vi "Autonomous Independent.vi"   [LabVIEW 2019]
doc: "This VI is called when autonomous begins, and will automatically be terminated when autonomous ends. You can carry out timed or sensor driven robot movement independently without needing to return to the caller."
uses:
  <vilib>/Rock Robotics/WPI/Utilities/WPI_GetSetVariantRefNum.vi
  Robot Global Data.vi
  <vilib>/Rock Robotics/Network Tables/NT Write Number.vi
  <vilib>/Rock Robotics/WPI/RobotDrive/WPI_RobotDriveArcadeDrive_Standard(NoSaturation).vi
  <vilib>/Rock Robotics/Network Tables/NT Write Numeric Array.vi
  <vilib>/Rock Robotics/Network Tables/NT Read String.vi
panel:
  # "Be sure to right-click and choose Data Operations>>Make Current Value default if you want to save the array values with the VI"
types:
  T1 = typedef "WPI_JoystickDevRef.ctl" = cluster{"Device":T2}
  T2 = typedef "WPI_JoystickDeviceEnum.ctl" = enum16{"USB 0", "USB 1", "USB 2", "USB 3", "USB 4", "USB 5"}
  T3 = typedef "WPI_RobotDriveDevRef.ctl" = cluster{"DevStatus":errorcluster, "Motors[]":T4[], "Square Inputs":bool, "Max Output":dbl}
  T4 = typedef "WPI_MotorControlDeviceRef.ctl" = cluster{"DeviceStatus":errorcluster, "Type":T5, "PWM":cluster{"PWM Channel":T6, "DeadBand":T7}, "CAN":cluster{"Device Number":u8, "SetOutput VI Ref":variant, "GetOutput VI Ref":variant, "Enable VI Ref":variant, "Disable VI Ref":variant, "Data":variant}, "Invert":bool, "DIO PWM":cluster{"PWM \"Enable\" Channel":T6, "DIOChannel":T8, "PWM Rate":dbl}}
  T5 = typedef "WPI_MotorControlType.ctl" = enum16{"PWM", "CAN", "DIO PWM"}
  T6 = typedef "FPGA_DIOPWMChannel.ctl" = enum8{"PWM 0", "PWM 1", "PWM 2", "PWM 3", "PWM 4", "PWM 5", "PWM 6", "PWM 7", "PWM 8", "PWM 9", "PWM MXP 0", "PWM MXP 1", "PWM MXP 2", "PWM MXP 3", "PWM MXP 4", "PWM MXP 5", "PWM MXP 6", "PWM MXP 7", "PWM MXP 8", "PWM MXP 9", "Invalid"}
  T7 = typedef "WPI_PWMDeadband.ctl" = cluster{"Name":string, "maxPositivePwm":i32, "minPositivePwm":i32, "centerPwm":i32, "maxNegativePwm":i32, "minNegativePwm":i32, "angularRange":u16}
  T8 = typedef "FPGA_DIOChannel.ctl" = enum8{"DIO 0", "DIO 1", "DIO 2", "DIO 3", "DIO 4", "DIO 5", "DIO 6", "DIO 7", "DIO 8", "DIO 9", "DIO MXP 0", "DIO MXP 1", "DIO MXP 2", "DIO MXP 3", "DIO MXP 4", "DIO MXP 5", "DIO MXP 6", "DIO MXP 7", "DIO MXP 8", "DIO MXP 9", "DIO MXP 10", "DIO MXP 11", "DIO MXP 12", "DIO MXP 13", "DIO MXP 14", "DIO MXP 15", "SPI Port CS1", "SPI Port CS2", "SPI Port CS3", "SPI Port MISO", "SPI Port MOSI", "Invalid"}
  T9 = typedef "WPI_ServoDeviceRef.ctl" = cluster{"DeviceStatus":errorcluster, "PWM Channel":T6, "DeadBand":T7}
  T10 = cluster{"RobotDriveDevRef":T3, "MotorControlDevRef":T4, "MotorControlDevRef":T4, "ServoDeviceRef":T9, "MotorControlDevRef":T4, "Distance":dbl}
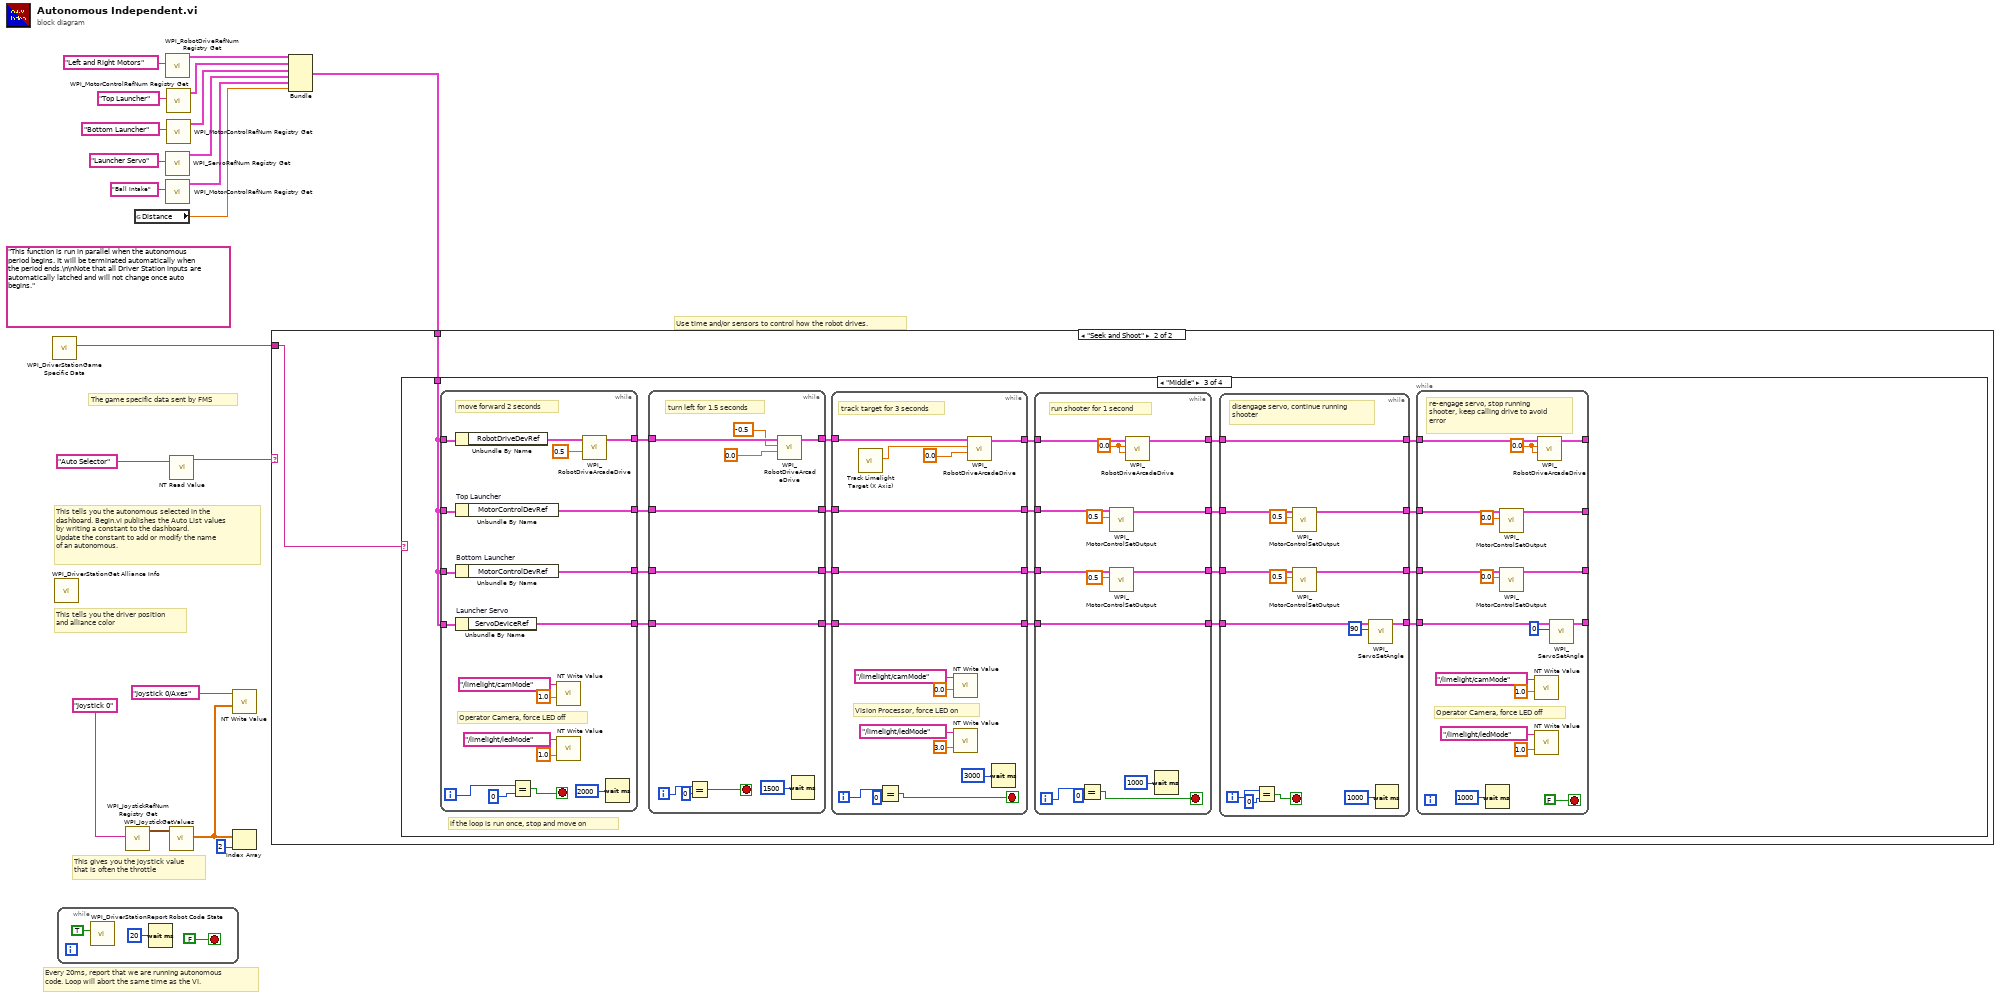
[diagram p0: block diagram]
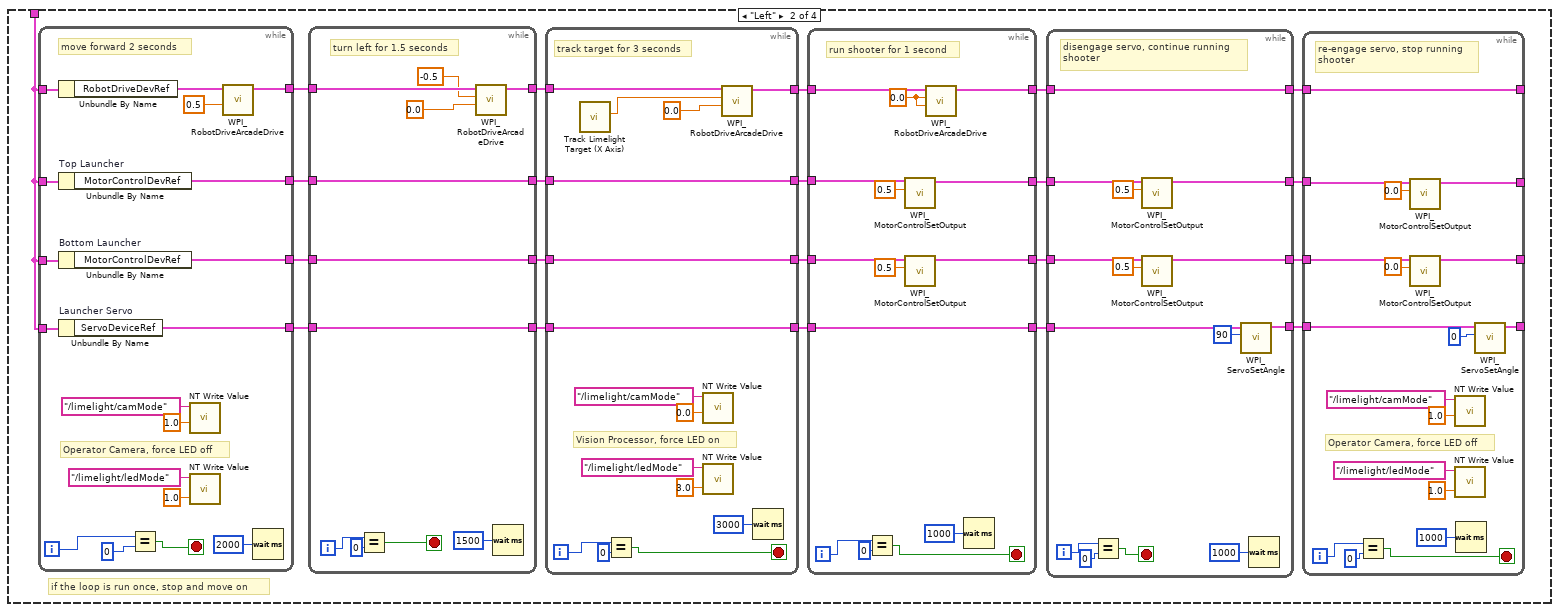
[diagram p4: hidden frame]
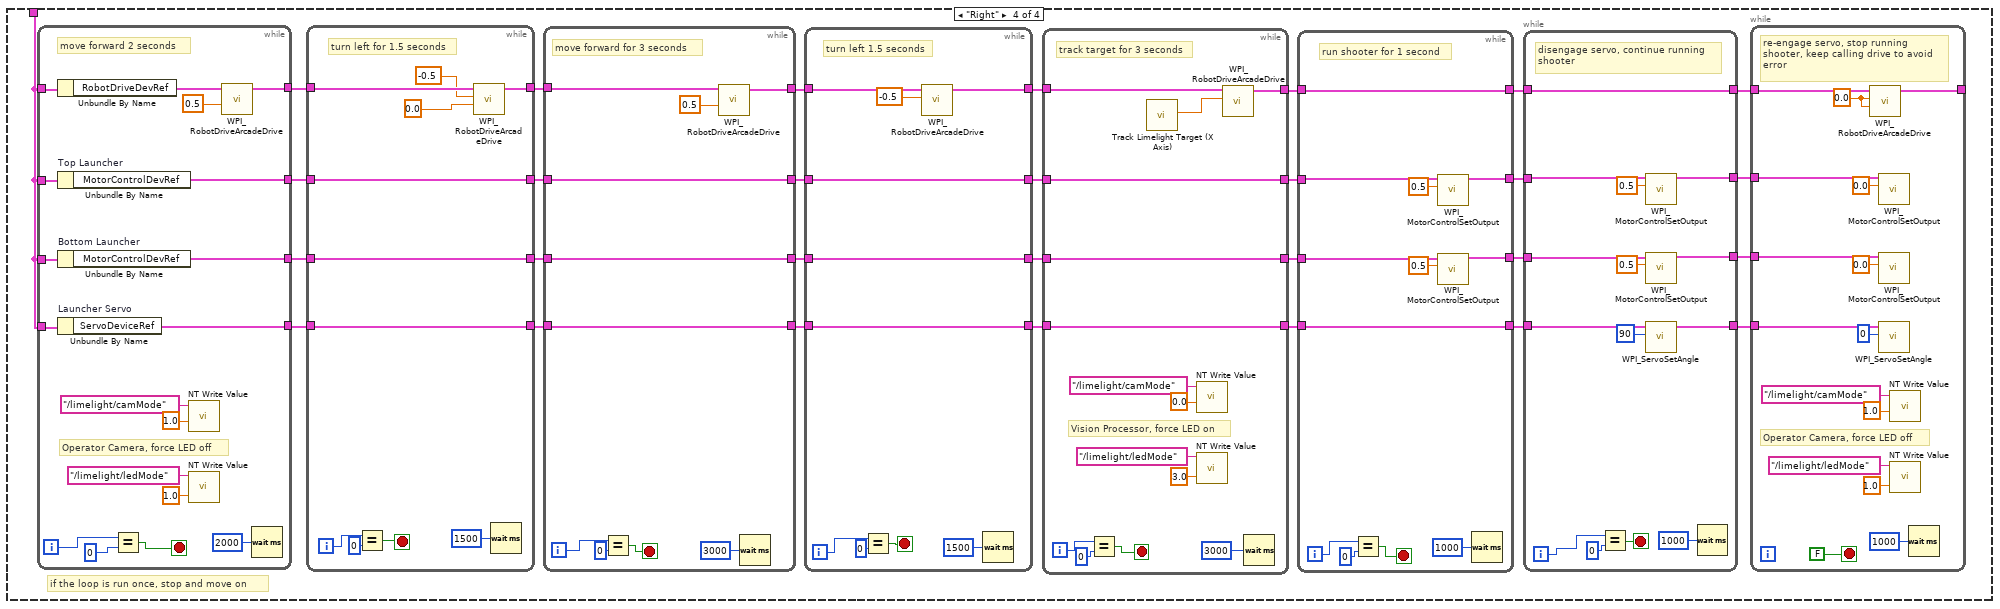
[diagram p5: hidden frame]
diagram:
  (unwired) "This function is run in parallel when the autonomous period begins. It will be terminated automatically when the period ends.\n\nNote that all Driver Station inputs are automatically latched and will not change once auto begins."
  # "The game specific data sent by FMS"
  # "This tells you the autonomous selected in the \ndashboard. Begin.vi publishes the Auto List values\nby writing a constant to the dashboard.\nUpdate the constant to add or modify the name\nof an autonomous."
  # "Every 20ms, report that we are running autonomous\ncode. Loop will abort the same time as the VI."
  # "This gives you the joystick value\nthat is often the throttle"
  # "Use time and/or sensors to control how the robot drives."
  # "This tells you the driver position\nand alliance color"
  n1 = call <vilib>:"WPI_DriverStationGame Specific Data.vi"() -> ("Game Specific Data"=w13:string)  [unwired: 11 in]
  n2 = call <vilib>:"WPI_DriverStationGet Alliance Info.vi"() -> ()  [unwired: 12 out]
  n3 = while {
    stop <- FALSE stop-if-true
    n4 = call <vilib>:"WPI_DriverStationReport Robot Code State.vi"("Autonomous"=TRUE) -> ()  [unwired: 10 in, 1 out]
    n5 = Wait (ms)(milliseconds to wait=u32 20) -> ()  [unwired: 1 out]
  }
  n6 = call <vilib>:"WPI_JoystickRefNum Registry Get.vi"("refnum name"="Joystick 0") -> ("JoystickDevRef"=w19:T1)  [unwired: 1 in, 9 out]
  n7 = global read "Robot Global Data.vi" "Distance"() -> (w2:dbl)
  n8 = call <vilib>:"WPI_RobotDriveRefNum Registry Get.vi"("refnum name"="Left and Right Motors") -> ("RobotDriveDevRef"=w11:T3)  [unwired: 9 in, 1 out]
  n9 = call <vilib>:"WPI_ServoRefNum Registry Get.vi"("refnum name"="Launcher Servo") -> ("ServoDeviceRef"=w5:T9)  [unwired: 9 in, 1 out]
  n10 = call <vilib>:"WPI_MotorControlRefNum Registry Get.vi"("refnum name"="Ball Intake") -> ("MotorControlDevRef"=w4:T4)  [unwired: 9 in, 1 out]
  n11 = call <vilib>:"WPI_MotorControlRefNum Registry Get.vi"("refnum name"="Top Launcher") -> ("MotorControlDevRef"=w8:T4)  [unwired: 9 in, 1 out]
  n12 = call <vilib>:"WPI_MotorControlRefNum Registry Get.vi"("refnum name"="Bottom Launcher") -> ("MotorControlDevRef"=w7:T4)  [unwired: 9 in, 1 out]
  n13 = call <vilib>:"WPI_JoystickGetValues.vi"("JoystickDevRef"=w19) -> ("Axes"=w15:dbl[])  [unwired: 6 in, 4 out]
  n14 = call-poly <vilib>:"NT Read Value.vi"("Name"="Auto Selector") -> ("String"=w16:string)  [unwired: 9 in, 1 out]
  n15 = call-poly <vilib>:"NT Write Value.vi"("Numeric Array"=w15, "Name"="Joystick 0/Axes") -> ()  [unwired: 9 in, 1 out]
  n16 = Index Array(array=w15, index=2) -> ()  [unwired: 1 out]
  n17 = Bundle("RobotDriveDevRef"=w11, "MotorControlDevRef"=w8, "MotorControlDevRef"=w7, "ServoDeviceRef"=w5, "MotorControlDevRef"=w4, "Distance"=w2) -> (w1:T10)  [unwired: 1 in]
  n18 = case shown="\"Seek and Shoot\"" w16 {
    tunnel: w13 -> [_ w24]
    tunnel: w1 -> [_ w25]
    frame Default {
      # "You can put your main auto here, or you can right-click on the case and make any\nother frame be the default case."
      # "This is the frame that will execute if no selection is made, or if it is not recognized"
    }
    frame "Seek and Shoot" {
      n19 = case shown="\"Middle\"" w24 {
        tunnel: w25 -> [_ w37 w148 w267]
        frame "", Default {
        }
        frame "Left" {
          # "if the loop is run once, stop and move on"
          n20 = while {
            tunnel: [w131] -> w46
            tunnel: w37 -> [w130]
            tunnel: w37 -> [w128]
            tunnel: w37 -> [w127]
            tunnel: [w126] -> w43
            tunnel: [w125] -> w40
            tunnel: w37 -> [w124]
            tunnel: [w123] -> w36
            i -> [w135]
            stop <- w133 stop-if-true
            # "Operator Camera, force LED off"
            # "move forward 2 seconds"
            n21 = Unbundle By Name(w130) -> ("RobotDriveDevRef"=w129:T3)
            n22 = Unbundle By Name "Top Launcher"(w128) -> ("MotorControlDevRef"=w126:T4)
            n23 = Unbundle By Name "Bottom Launcher"(w127) -> ("MotorControlDevRef"=w125:T4)
            n24 = Unbundle By Name "Launcher Servo"(w124) -> ("ServoDeviceRef"=w123:T9)
            n25 = Equal?(x=w135, y=0) -> (x = y?=w133:bool)
            n26 = call-poly <vilib>:"NT Write Value.vi"("Numeric"=1.0, "Name"="/limelight/camMode") -> ()  [unwired: 9 in, 1 out]
            n27 = call-poly <vilib>:"NT Write Value.vi"("Numeric"=1.0, "Name"="/limelight/ledMode") -> ()  [unwired: 9 in, 1 out]
            n28 = call-poly <vilib>:"WPI_RobotDriveArcadeDrive.vi"("Y axis value"=0.5, "RobotDriveDevRef"=w129) -> ("RobotDriveDevRef"=w131:T3)  [unwired: 7 in, 2 out]
            n29 = Wait (ms)(milliseconds to wait=u32 2000) -> ()  [unwired: 1 out]
          }
          n30 = while {
            tunnel: w46 -> [w118]
            tunnel: [w111] -> w45
            tunnel: w43 -> [w110]
            tunnel: [w110] -> w42
            tunnel: w40 -> [w109]
            tunnel: [w109] -> w39
            tunnel: w36 -> [w108]
            tunnel: [w108] -> w35
            i -> [w114]
            stop <- w112 stop-if-true
            # "turn left for 1.5 seconds"
            n31 = Equal?(x=w114, y=0) -> (x = y?=w112:bool)
            n32 = call-poly <vilib>:"WPI_RobotDriveArcadeDrive.vi"("Y axis value"=0.0, "X axis value"=-0.5, "RobotDriveDevRef"=w118) -> ("RobotDriveDevRef"=w111:T3)  [unwired: 6 in, 2 out]
            n33 = Wait (ms)(milliseconds to wait=u32 1500) -> ()  [unwired: 1 out]
          }
          n34 = while {
            tunnel: w45 -> [w107]
            tunnel: [w100] -> w44
            tunnel: w42 -> [w99]
            tunnel: [w99] -> w41
            tunnel: w39 -> [w98]
            tunnel: [w98] -> w38
            tunnel: w35 -> [w97]
            tunnel: [w97] -> w34
            i -> [w102]
            stop <- w101 stop-if-true
            # "Vision Processor, force LED on"
            # "track target for 3 seconds"
            n35 = call "Track Limelight Target (X Axis).vi"() -> ("Joystick X"=w106:dbl)  [unwired: 11 in]
            n36 = Equal?(x=w102, y=0) -> (x = y?=w101:bool)
            n37 = call-poly <vilib>:"NT Write Value.vi"("Numeric"=0.0, "Name"="/limelight/camMode") -> ()  [unwired: 9 in, 1 out]
            n38 = call-poly <vilib>:"NT Write Value.vi"("Numeric"=3.0, "Name"="/limelight/ledMode") -> ()  [unwired: 9 in, 1 out]
            n39 = call-poly <vilib>:"WPI_RobotDriveArcadeDrive.vi"("Y axis value"=0.0, "X axis value"=w106, "RobotDriveDevRef"=w107) -> ("RobotDriveDevRef"=w100:T3)  [unwired: 6 in, 2 out]
            n40 = Wait (ms)(milliseconds to wait=u32 3000) -> ()  [unwired: 1 out]
          }
          n41 = while {
            tunnel: w44 -> [w92]
            tunnel: w41 -> [w89]
            tunnel: w38 -> [w90]
            tunnel: [w86] -> w31
            tunnel: [w85] -> w32
            tunnel: w34 -> [w80]
            tunnel: [w80] -> w33
            tunnel: [w79] -> w30
            i -> [w83]
            stop <- w82 stop-if-true
            w91 = 0.0 ("X axis value")
            # "run shooter for 1 second"
            n42 = Equal?(x=w83, y=0) -> (x = y?=w82:bool)
            n43 = call <vilib>:"WPI_MotorControlSetOutput.vi"("Output"=0.5, "MotorControlDevRef"=w89) -> ("MotorControlDevRef"=w85:T4)  [unwired: 7 in, 2 out]
            n44 = call <vilib>:"WPI_MotorControlSetOutput.vi"("Output"=0.5, "MotorControlDevRef"=w90) -> ("MotorControlDevRef"=w86:T4)  [unwired: 7 in, 2 out]
            n45 = call-poly <vilib>:"WPI_RobotDriveArcadeDrive.vi"("Y axis value"=w91, "X axis value"=w91, "RobotDriveDevRef"=w92) -> ("RobotDriveDevRef"=w79:T3)  [unwired: 6 in, 2 out]
            n46 = Wait (ms)(milliseconds to wait=u32 1000) -> ()  [unwired: 1 out]
          }
          n47 = while {
            tunnel: w33 -> [w74]
            tunnel: [w73] -> w29
            tunnel: w32 -> [w71]
            tunnel: w31 -> [w69]
            tunnel: [w68] -> w28
            tunnel: [w67] -> w27
            tunnel: w30 -> [w65]
            tunnel: [w65] -> w26
            i -> [w77]
            stop <- w75 stop-if-true
            # "disengage servo, continue running\nshooter"
            n48 = Equal?(x=w77, y=0) -> (x = y?=w75:bool)
            n49 = call <vilib>:"WPI_MotorControlSetOutput.vi"("Output"=0.5, "MotorControlDevRef"=w71) -> ("MotorControlDevRef"=w68:T4)  [unwired: 7 in, 2 out]
            n50 = call <vilib>:"WPI_MotorControlSetOutput.vi"("Output"=0.5, "MotorControlDevRef"=w69) -> ("MotorControlDevRef"=w67:T4)  [unwired: 7 in, 2 out]
            n51 = call <vilib>:"WPI_ServoSetAngle.vi"("Angle"=90, "ServoDeviceRef"=w74) -> ("ServoDeviceRef"=w73:T9)  [unwired: 8 in, 1 out]
            n52 = Wait (ms)(milliseconds to wait=u32 1000) -> ()  [unwired: 1 out]
          }
          n53 = while {
            tunnel: w29 -> [w60]
            tunnel: [w59] -> _
            tunnel: w28 -> [w55]
            tunnel: w27 -> [w54]
            tunnel: [w53] -> _
            tunnel: [w52] -> _
            tunnel: w26 -> [w51]
            tunnel: [w51] -> _
            i -> [w63]
            stop <- w62 stop-if-true
            # "Operator Camera, force LED off"
            # "re-engage servo, stop running\nshooter"
            n54 = Equal?(x=w63, y=0) -> (x = y?=w62:bool)
            n55 = call <vilib>:"WPI_MotorControlSetOutput.vi"("Output"=0.0, "MotorControlDevRef"=w55) -> ("MotorControlDevRef"=w52:T4)  [unwired: 7 in, 2 out]
            n56 = call <vilib>:"WPI_MotorControlSetOutput.vi"("Output"=0.0, "MotorControlDevRef"=w54) -> ("MotorControlDevRef"=w53:T4)  [unwired: 7 in, 2 out]
            n57 = call-poly <vilib>:"NT Write Value.vi"("Numeric"=1.0, "Name"="/limelight/camMode") -> ()  [unwired: 9 in, 1 out]
            n58 = call-poly <vilib>:"NT Write Value.vi"("Numeric"=1.0, "Name"="/limelight/ledMode") -> ()  [unwired: 9 in, 1 out]
            n59 = Wait (ms)(milliseconds to wait=u32 1000) -> ()  [unwired: 1 out]
            n60 = call <vilib>:"WPI_ServoSetAngle.vi"("Angle"=0, "ServoDeviceRef"=w60) -> ("ServoDeviceRef"=w59:T9)  [unwired: 8 in, 1 out]
          }
        }
        frame "Middle" {
          # "if the loop is run once, stop and move on"
          n61 = while {
            tunnel: [w242] -> w157
            tunnel: w148 -> [w241]
            tunnel: w148 -> [w239]
            tunnel: w148 -> [w238]
            tunnel: [w237] -> w154
            tunnel: [w236] -> w151
            tunnel: w148 -> [w235]
            tunnel: [w234] -> w147
            i -> [w246]
            stop <- w244 stop-if-true
            # "Operator Camera, force LED off"
            # "move forward 2 seconds"
            n62 = Unbundle By Name(w241) -> ("RobotDriveDevRef"=w240:T3)
            n63 = Unbundle By Name "Top Launcher"(w239) -> ("MotorControlDevRef"=w237:T4)
            n64 = Unbundle By Name "Bottom Launcher"(w238) -> ("MotorControlDevRef"=w236:T4)
            n65 = Unbundle By Name "Launcher Servo"(w235) -> ("ServoDeviceRef"=w234:T9)
            n66 = Equal?(x=w246, y=0) -> (x = y?=w244:bool)
            n67 = call-poly <vilib>:"NT Write Value.vi"("Numeric"=1.0, "Name"="/limelight/camMode") -> ()  [unwired: 9 in, 1 out]
            n68 = call-poly <vilib>:"NT Write Value.vi"("Numeric"=1.0, "Name"="/limelight/ledMode") -> ()  [unwired: 9 in, 1 out]
            n69 = call-poly <vilib>:"WPI_RobotDriveArcadeDrive.vi"("Y axis value"=0.5, "RobotDriveDevRef"=w240) -> ("RobotDriveDevRef"=w242:T3)  [unwired: 7 in, 2 out]
            n70 = Wait (ms)(milliseconds to wait=u32 2000) -> ()  [unwired: 1 out]
          }
          n71 = while {
            tunnel: w157 -> [w229]
            tunnel: [w222] -> w156
            tunnel: w154 -> [w221]
            tunnel: [w221] -> w153
            tunnel: w151 -> [w220]
            tunnel: [w220] -> w150
            tunnel: w147 -> [w219]
            tunnel: [w219] -> w146
            i -> [w225]
            stop <- w223 stop-if-true
            # "turn left for 1.5 seconds"
            n72 = Equal?(x=w225, y=0) -> (x = y?=w223:bool)
            n73 = call-poly <vilib>:"WPI_RobotDriveArcadeDrive.vi"("Y axis value"=0.0, "X axis value"=-0.5, "RobotDriveDevRef"=w229) -> ("RobotDriveDevRef"=w222:T3)  [unwired: 6 in, 2 out]
            n74 = Wait (ms)(milliseconds to wait=u32 1500) -> ()  [unwired: 1 out]
          }
          n75 = while {
            tunnel: w156 -> [w218]
            tunnel: [w211] -> w155
            tunnel: w153 -> [w210]
            tunnel: [w210] -> w152
            tunnel: w150 -> [w209]
            tunnel: [w209] -> w149
            tunnel: w146 -> [w208]
            tunnel: [w208] -> w145
            i -> [w213]
            stop <- w212 stop-if-true
            # "Vision Processor, force LED on"
            # "track target for 3 seconds"
            n76 = call "Track Limelight Target (X Axis).vi"() -> ("Joystick X"=w217:dbl)  [unwired: 11 in]
            n77 = Equal?(x=w213, y=0) -> (x = y?=w212:bool)
            n78 = call-poly <vilib>:"NT Write Value.vi"("Numeric"=0.0, "Name"="/limelight/camMode") -> ()  [unwired: 9 in, 1 out]
            n79 = call-poly <vilib>:"NT Write Value.vi"("Numeric"=3.0, "Name"="/limelight/ledMode") -> ()  [unwired: 9 in, 1 out]
            n80 = call-poly <vilib>:"WPI_RobotDriveArcadeDrive.vi"("Y axis value"=0.0, "X axis value"=w217, "RobotDriveDevRef"=w218) -> ("RobotDriveDevRef"=w211:T3)  [unwired: 6 in, 2 out]
            n81 = Wait (ms)(milliseconds to wait=u32 3000) -> ()  [unwired: 1 out]
          }
          n82 = while {
            tunnel: w155 -> [w203]
            tunnel: w152 -> [w200]
            tunnel: w149 -> [w201]
            tunnel: [w197] -> w142
            tunnel: [w196] -> w143
            tunnel: w145 -> [w191]
            tunnel: [w191] -> w144
            tunnel: [w190] -> w141
            i -> [w194]
            stop <- w193 stop-if-true
            w202 = 0.0 ("X axis value")
            # "run shooter for 1 second"
            n83 = Equal?(x=w194, y=0) -> (x = y?=w193:bool)
            n84 = call <vilib>:"WPI_MotorControlSetOutput.vi"("Output"=0.5, "MotorControlDevRef"=w200) -> ("MotorControlDevRef"=w196:T4)  [unwired: 7 in, 2 out]
            n85 = call <vilib>:"WPI_MotorControlSetOutput.vi"("Output"=0.5, "MotorControlDevRef"=w201) -> ("MotorControlDevRef"=w197:T4)  [unwired: 7 in, 2 out]
            n86 = call-poly <vilib>:"WPI_RobotDriveArcadeDrive.vi"("Y axis value"=w202, "X axis value"=w202, "RobotDriveDevRef"=w203) -> ("RobotDriveDevRef"=w190:T3)  [unwired: 6 in, 2 out]
            n87 = Wait (ms)(milliseconds to wait=u32 1000) -> ()  [unwired: 1 out]
          }
          n88 = while {
            tunnel: w144 -> [w185]
            tunnel: [w184] -> w140
            tunnel: w143 -> [w182]
            tunnel: w142 -> [w180]
            tunnel: [w179] -> w139
            tunnel: [w178] -> w138
            tunnel: w141 -> [w176]
            tunnel: [w176] -> w137
            i -> [w188]
            stop <- w186 stop-if-true
            # "disengage servo, continue running\nshooter"
            n89 = Equal?(x=w188, y=0) -> (x = y?=w186:bool)
            n90 = call <vilib>:"WPI_MotorControlSetOutput.vi"("Output"=0.5, "MotorControlDevRef"=w182) -> ("MotorControlDevRef"=w179:T4)  [unwired: 7 in, 2 out]
            n91 = call <vilib>:"WPI_MotorControlSetOutput.vi"("Output"=0.5, "MotorControlDevRef"=w180) -> ("MotorControlDevRef"=w178:T4)  [unwired: 7 in, 2 out]
            n92 = call <vilib>:"WPI_ServoSetAngle.vi"("Angle"=90, "ServoDeviceRef"=w185) -> ("ServoDeviceRef"=w184:T9)  [unwired: 8 in, 1 out]
            n93 = Wait (ms)(milliseconds to wait=u32 1000) -> ()  [unwired: 1 out]
          }
          n94 = while {
            tunnel: w140 -> [w174]
            tunnel: [w173] -> _
            tunnel: w139 -> [w169]
            tunnel: w138 -> [w168]
            tunnel: [w167] -> _
            tunnel: [w166] -> _
            tunnel: w137 -> [w160]
            tunnel: [w159] -> _
            stop <- FALSE stop-if-true
            w158 = 0.0 ("X axis value")
            # "Operator Camera, force LED off"
            # "re-engage servo, stop running\nshooter, keep calling drive to avoid\nerror"
            n95 = Wait (ms)(milliseconds to wait=u32 1000) -> ()  [unwired: 1 out]
            n96 = call <vilib>:"WPI_MotorControlSetOutput.vi"("Output"=0.0, "MotorControlDevRef"=w169) -> ("MotorControlDevRef"=w166:T4)  [unwired: 7 in, 2 out]
            n97 = call <vilib>:"WPI_MotorControlSetOutput.vi"("Output"=0.0, "MotorControlDevRef"=w168) -> ("MotorControlDevRef"=w167:T4)  [unwired: 7 in, 2 out]
            n98 = call-poly <vilib>:"NT Write Value.vi"("Numeric"=1.0, "Name"="/limelight/camMode") -> ()  [unwired: 9 in, 1 out]
            n99 = call-poly <vilib>:"NT Write Value.vi"("Numeric"=1.0, "Name"="/limelight/ledMode") -> ()  [unwired: 9 in, 1 out]
            n100 = call-poly <vilib>:"WPI_RobotDriveArcadeDrive.vi"("Y axis value"=w158, "X axis value"=w158, "RobotDriveDevRef"=w160) -> ("RobotDriveDevRef"=w159:T3)  [unwired: 6 in, 2 out]
            n101 = call <vilib>:"WPI_ServoSetAngle.vi"("Angle"=0, "ServoDeviceRef"=w174) -> ("ServoDeviceRef"=w173:T9)  [unwired: 8 in, 1 out]
          }
        }
        frame "Right" {
          # "if the loop is run once, stop and move on"
          n102 = while {
            tunnel: [w375] -> w276
            tunnel: w267 -> [w374]
            tunnel: w267 -> [w372]
            tunnel: w267 -> [w371]
            tunnel: [w370] -> w273
            tunnel: [w369] -> w270
            tunnel: w267 -> [w368]
            tunnel: [w367] -> w266
            i -> [w379]
            stop <- w377 stop-if-true
            # "Operator Camera, force LED off"
            # "move forward 2 seconds"
            n103 = Unbundle By Name(w374) -> ("RobotDriveDevRef"=w373:T3)
            n104 = Unbundle By Name "Top Launcher"(w372) -> ("MotorControlDevRef"=w370:T4)
            n105 = Unbundle By Name "Bottom Launcher"(w371) -> ("MotorControlDevRef"=w369:T4)
            n106 = Unbundle By Name "Launcher Servo"(w368) -> ("ServoDeviceRef"=w367:T9)
            n107 = Equal?(x=w379, y=0) -> (x = y?=w377:bool)
            n108 = call-poly <vilib>:"NT Write Value.vi"("Numeric"=1.0, "Name"="/limelight/camMode") -> ()  [unwired: 9 in, 1 out]
            n109 = call-poly <vilib>:"NT Write Value.vi"("Numeric"=1.0, "Name"="/limelight/ledMode") -> ()  [unwired: 9 in, 1 out]
            n110 = call-poly <vilib>:"WPI_RobotDriveArcadeDrive.vi"("Y axis value"=0.5, "RobotDriveDevRef"=w373) -> ("RobotDriveDevRef"=w375:T3)  [unwired: 7 in, 2 out]
            n111 = Wait (ms)(milliseconds to wait=u32 2000) -> ()  [unwired: 1 out]
          }
          n112 = while {
            tunnel: w276 -> [w362]
            tunnel: [w355] -> w275
            tunnel: w273 -> [w354]
            tunnel: [w354] -> w272
            tunnel: w270 -> [w353]
            tunnel: [w353] -> w269
            tunnel: w266 -> [w352]
            tunnel: [w352] -> w265
            i -> [w358]
            stop <- w356 stop-if-true
            # "turn left for 1.5 seconds"
            n113 = Equal?(x=w358, y=0) -> (x = y?=w356:bool)
            n114 = call-poly <vilib>:"WPI_RobotDriveArcadeDrive.vi"("Y axis value"=0.0, "X axis value"=-0.5, "RobotDriveDevRef"=w362) -> ("RobotDriveDevRef"=w355:T3)  [unwired: 6 in, 2 out]
            n115 = Wait (ms)(milliseconds to wait=u32 1500) -> ()  [unwired: 1 out]
          }
          n116 = while {
            tunnel: w275 -> [w351]
            tunnel: [w346] -> w274
            tunnel: w272 -> [w345]
            tunnel: [w345] -> w271
            tunnel: w269 -> [w344]
            tunnel: [w344] -> w268
            tunnel: w265 -> [w343]
            tunnel: [w343] -> w264
            i -> [w348]
            stop <- w347 stop-if-true
            # "move forward for 3 seconds"
            n117 = Equal?(x=w348, y=0) -> (x = y?=w347:bool)
            n118 = call-poly <vilib>:"WPI_RobotDriveArcadeDrive.vi"("Y axis value"=0.5, "RobotDriveDevRef"=w351) -> ("RobotDriveDevRef"=w346:T3)  [unwired: 7 in, 2 out]
            n119 = Wait (ms)(milliseconds to wait=u32 3000) -> ()  [unwired: 1 out]
          }
          n120 = while {
            tunnel: w274 -> [w341]
            tunnel: w271 -> [w332]
            tunnel: w268 -> [w333]
            tunnel: w264 -> [w335]
            tunnel: [w335] -> w263
            tunnel: [w334] -> w262
            tunnel: [w333] -> w261
            tunnel: [w332] -> w260
            i -> [w338]
            stop <- w337 stop-if-true
            # "turn left 1.5 seconds"
            n121 = Equal?(x=w338, y=0) -> (x = y?=w337:bool)
            n122 = call-poly <vilib>:"WPI_RobotDriveArcadeDrive.vi"("X axis value"=-0.5, "RobotDriveDevRef"=w341) -> ("RobotDriveDevRef"=w334:T3)  [unwired: 7 in, 2 out]
            n123 = Wait (ms)(milliseconds to wait=u32 1500) -> ()  [unwired: 1 out]
          }
          n124 = while {
            tunnel: w263 -> [w327]
            tunnel: w262 -> [w324]
            tunnel: w261 -> [w326]
            tunnel: w260 -> [w325]
            tunnel: [w327] -> w259
            tunnel: [w326] -> w258
            tunnel: [w325] -> w257
            tunnel: [w323] -> w256
            i -> [w330]
            stop <- w328 stop-if-true
            # "Vision Processor, force LED on"
            # "track target for 3 seconds"
            n125 = Equal?(x=w330, y=0) -> (x = y?=w328:bool)
            n126 = call "Track Limelight Target (X Axis).vi"() -> ("Joystick X"=w322:dbl)  [unwired: 11 in]
            n127 = call-poly <vilib>:"NT Write Value.vi"("Numeric"=0.0, "Name"="/limelight/camMode") -> ()  [unwired: 9 in, 1 out]
            n128 = call-poly <vilib>:"NT Write Value.vi"("Numeric"=3.0, "Name"="/limelight/ledMode") -> ()  [unwired: 9 in, 1 out]
            n129 = call-poly <vilib>:"WPI_RobotDriveArcadeDrive.vi"("X axis value"=w322, "RobotDriveDevRef"=w324) -> ("RobotDriveDevRef"=w323:T3)  [unwired: 7 in, 2 out]
            n130 = Wait (ms)(milliseconds to wait=u32 3000) -> ()  [unwired: 1 out]
          }
          n131 = while {
            tunnel: w259 -> [w306]
            tunnel: w258 -> [w312]
            tunnel: w257 -> [w311]
            tunnel: w256 -> [w313]
            tunnel: [w313] -> w252
            tunnel: [w310] -> w255
            tunnel: [w309] -> w254
            tunnel: [w306] -> w253
            i -> [w316]
            stop <- w314 stop-if-true
            # "run shooter for 1 second"
            n132 = Equal?(x=w316, y=0) -> (x = y?=w314:bool)
            n133 = call <vilib>:"WPI_MotorControlSetOutput.vi"("Output"=0.5, "MotorControlDevRef"=w311) -> ("MotorControlDevRef"=w310:T4)  [unwired: 7 in, 2 out]
            n134 = call <vilib>:"WPI_MotorControlSetOutput.vi"("Output"=0.5, "MotorControlDevRef"=w312) -> ("MotorControlDevRef"=w309:T4)  [unwired: 7 in, 2 out]
            n135 = Wait (ms)(milliseconds to wait=u32 1000) -> ()  [unwired: 1 out]
          }
          n136 = while {
            tunnel: w255 -> [w300]
            tunnel: w254 -> [w299]
            tunnel: w253 -> [w298]
            tunnel: w252 -> [w296]
            tunnel: [w296] -> w248
            tunnel: [w294] -> w251
            tunnel: [w293] -> w250
            tunnel: [w292] -> w249
            i -> [w304]
            stop <- w303 stop-if-true
            # "disengage servo, continue running\nshooter"
            n137 = Equal?(x=w304, y=0) -> (x = y?=w303:bool)
            n138 = call <vilib>:"WPI_MotorControlSetOutput.vi"("Output"=0.5, "MotorControlDevRef"=w300) -> ("MotorControlDevRef"=w294:T4)  [unwired: 7 in, 2 out]
            n139 = call <vilib>:"WPI_MotorControlSetOutput.vi"("Output"=0.5, "MotorControlDevRef"=w299) -> ("MotorControlDevRef"=w293:T4)  [unwired: 7 in, 2 out]
            n140 = call <vilib>:"WPI_ServoSetAngle.vi"("Angle"=90, "ServoDeviceRef"=w298) -> ("ServoDeviceRef"=w292:T9)  [unwired: 8 in, 1 out]
            n141 = Wait (ms)(milliseconds to wait=u32 1000) -> ()  [unwired: 1 out]
          }
          n142 = while {
            tunnel: w251 -> [w287]
            tunnel: w250 -> [w286]
            tunnel: w249 -> [w285]
            tunnel: w248 -> [w279]
            tunnel: [w277] -> _
            stop <- FALSE stop-if-true
            w278 = 0.0 ("X axis value")
            # "Operator Camera, force LED off"
            # "re-engage servo, stop running\nshooter, keep calling drive to avoid\nerror"
            n143 = call-poly <vilib>:"WPI_RobotDriveArcadeDrive.vi"("Y axis value"=w278, "X axis value"=w278, "RobotDriveDevRef"=w279) -> ("RobotDriveDevRef"=w277:T3)  [unwired: 6 in, 2 out]
            n144 = call <vilib>:"WPI_MotorControlSetOutput.vi"("Output"=0.0, "MotorControlDevRef"=w287) -> ()  [unwired: 7 in, 3 out]
            n145 = call <vilib>:"WPI_MotorControlSetOutput.vi"("Output"=0.0, "MotorControlDevRef"=w286) -> ()  [unwired: 7 in, 3 out]
            n146 = call <vilib>:"WPI_ServoSetAngle.vi"("Angle"=0, "ServoDeviceRef"=w285) -> ()  [unwired: 8 in, 2 out]
            n147 = call-poly <vilib>:"NT Write Value.vi"("Numeric"=1.0, "Name"="/limelight/camMode") -> ()  [unwired: 9 in, 1 out]
            n148 = call-poly <vilib>:"NT Write Value.vi"("Numeric"=1.0, "Name"="/limelight/ledMode") -> ()  [unwired: 9 in, 1 out]
            n149 = Wait (ms)(milliseconds to wait=u32 1000) -> ()  [unwired: 1 out]
          }
        }
      }
    }
  }
